vi "Arduino Read Raw String.vi"(8 "error in (no error)":errorcluster, 11 "FW Arduino Control in":refnum<class "FW Arduino Control.lvclass">) -> (0 "error out":errorcluster, 2 "Raw String":string, 3 "FW Arduino Control out":refnum<class "FW Arduino Control.lvclass">)   [LabVIEW 2022 SP3, in "FW Arduino Control.lvclass"]
uses:
  FW Arduino Control.lvclass
  Filter Wheel Object/Filter Wheel.lvclass
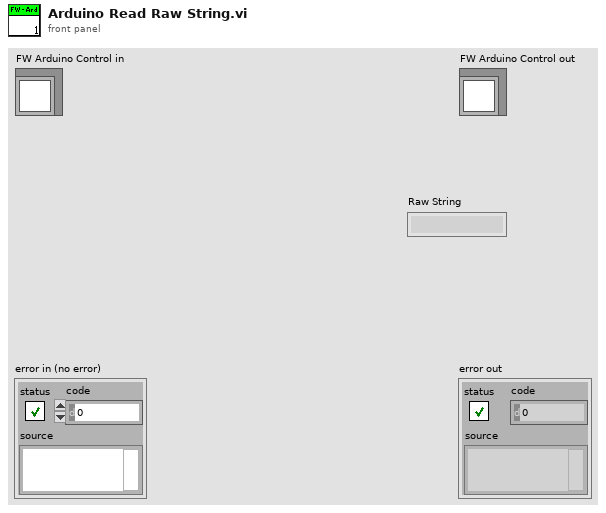
[diagram p1: front panel]
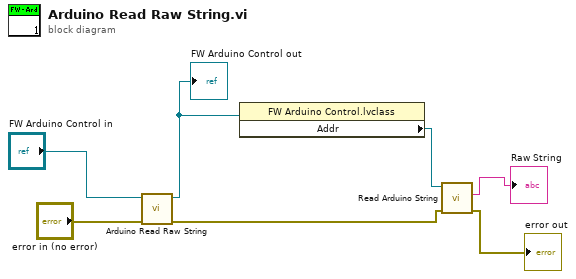
[diagram p0: block diagram]
diagram:
  n1 = call-parent "Arduino Read Raw String.vi"("error in (no error)"="error in (no error)", "Filter Wheel in"="FW Arduino Control in") -> ("error out"=w2:errorcluster, "Filter Wheel out"=w4:refnum<class "FW Arduino Control.lvclass">)  [unwired: 7 in, 1 out]
  "FW Arduino Control out" <- w4
  n2 = property class="FW Arduino Control.lvclass"(reference=w4) -> ("Addr"=w3:refnum<visa-resource-name>)  [unwired: 1 in, 2 out]
  n3 = call "Read Arduino String.vi"("error in (no error)"=w2, "reference"=w3) -> ("error out"=→"error out":errorcluster, "response"=→"Raw String":string)  [unwired: 7 in, 1 out]
